vi "Check Plugin Visibility.vi"(8 "error in (no error)":errorcluster, 11 "GUI Manager Module in":refnum<class "GUI Manager Module.lvclass">) -> (0 "error out":errorcluster, 3 "GUI Manager Module out":refnum<class "GUI Manager Module.lvclass">)   [LabVIEW 2020, in "VolatusGUI.lvlib" / "GUI Manager Module.lvclass"]
uses:
  GUI Manager Module.lvclass
  C:/dev/lv20CE/relink/lv-volatus/Volatus/Module/Module.lvclass
  GUI Manager Module.lvclass/GUI Manager Module.ctl
  Volatus/Module/Module.lvclass/Module.ctl
  Volatus/MessageQ/MessageQ.lvclass/MessageQ.ctl
  Volatus/Module/Self Q.vi
  Volatus/MessageQ/Send.vi
  Volatus/Module/Module.lvclass
  C:/dev/lv20CE/relink/lv-volatus/VolatusGUI/GUI Manager Module/GUI Manager Module.lvclass
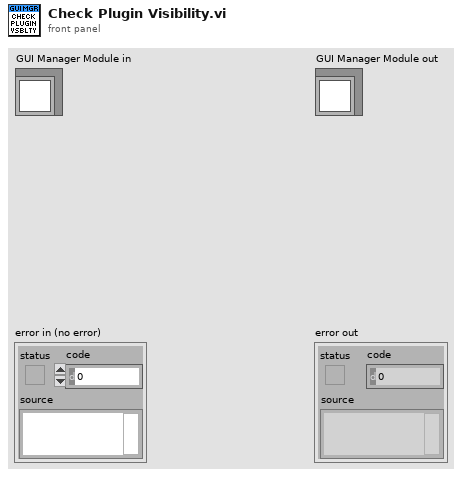
[diagram p1: front panel]
types:
  T1 = typedef "VolatusGUI.lvlib/GUI State.ctl" = cluster{"GUI ID":string, "Visible":bool, "Visibility Set":bool, "Bounds":T2, "Bounds Set":bool}
  T2 = typedef "LVRectTypeDef.ctl" = cluster{"Left":i16, "Top":i16, "Right":i16, "Bottom":i16}
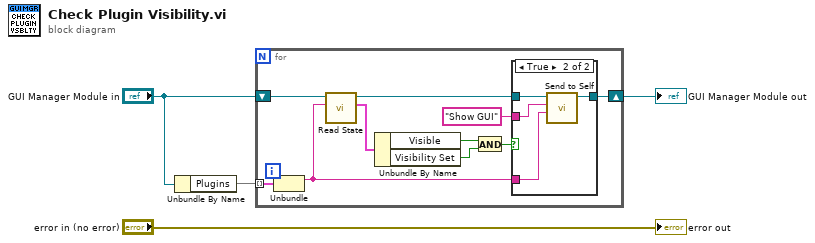
[diagram p0: block diagram]
diagram:
  n1 = Unbundle By Name("GUI Manager Module in") -> ("Plugins"=w1:map{string, path})
  n2 = for {
    shift-right: [w5] -> w2
    shift-left: "GUI Manager Module in" -> [w13]
    tunnel: w1 -> [w14] mode=indexing
    n3 = Unbundle(w14) -> (w6:string)  [unwired: 1 out]
    n4 = call "Read State.vi"("GUI ID"=w6, "GUI Manager Module in"=w13) -> ("GUI State"=w12:T1, "GUI Manager Module out"=w9:refnum<class "GUI Manager Module.lvclass">)  [unwired: 7 in, 1 out]
    n5 = Unbundle By Name(w12) -> ("Visible"=w11:bool, "Visibility Set"=w10:bool)
    n6 = And(x=w11, y=w10) -> (x .and. y?=w8:bool)
    n7 = case shown="True" w8 {
      tunnel: w9 -> [w15 w19]
      tunnel: "Show GUI" ("ID") -> [_ w18]
      tunnel: w6 -> [_ w17]
      tunnel: [w15 w16] -> w5
      frame False {
      }
      frame True {
        n8 = call "Send to Self.vi"("Data"=w17, "Message ID"=w18, "Module in"=w19) -> ("Module in"=w16:refnum<class "GUI Manager Module.lvclass">)  [unwired: 7 in, 1 out]
      }
    }
  }
  "GUI Manager Module out" <- w2
  "error out" <- "error in (no error)"
